vi "PH_Cam_BaseClass.save Image.vi"(0 "i ref in":refnum<vi>, 5 "error in (no error)":errorcluster) -> (14 "i ref out":refnum<vi>, 19 "error out":errorcluster)   [LabVIEW 2014, in "PH_Cam_BaseClass.lvlib"]
doc: "This CI saves the cam image if it finds a valid file refnum in own attributes."
uses:
  PH_Cam_BaseClass.lvlib
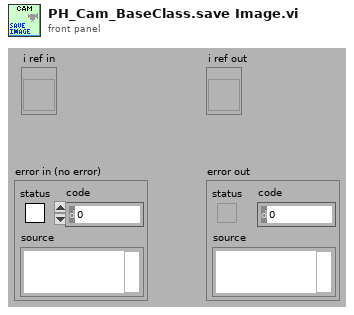
[diagram p1: front panel]
types:
  T1 = typedef "PH_Cam_BaseClass.lvlib/PH_Cam_BaseClass.i attribute.ctl" = cluster{"Gui Refs":T2, "Cam":cluster{"Source Notifier":refnum<notifier>, "Error":errorcluster, "Camera ID":string}, "Images":cluster{"Cam":T3, "Operation":T3, "PSDB":T3}, "Window Image":cluster{"Indicate Image":bool, "Window No.":i32, "Scale Facor":dbl, "Center Cross":bool, "Subtract Backgr":bool, "CoG":bool, "Color Palette":cluster{"Red":u8, "Green":u8, "Blue":u8}[], "Image On":bool}, "Default Prdc Int":i32, "Performance":cluster{"on":bool, "Timestamp Last Frame":i32}, "Histogram":cluster{"on":bool, "Mapping":bool}, "Save Image":cluster{"Save":bool, "File refnum":refnum<file>}, "Setting Service ID":i32, "Screen":cluster{"x-resolution":i16, "y-resolution":i16}, "On":bool, "Constructor finished":bool, "configured":bool}
  T2 = typedef "PH_Cam_BaseClass.lvlib/PH_Cam_BaseClass.GUI Refs.ctl" = cluster{"Frame Rate":refnum<vi>, "Get Frame Rate":refnum<vi>, "Show Image":refnum<vi>, "Get Histogram":refnum<vi>, "Mapping":refnum<vi>, "Histogram":refnum<vi>, "Center Cross":refnum<vi>, "Center of Gravity":refnum<vi>, "Scale Factor [%]":refnum<vi>, "Save Image":refnum<vi>, "Palette":refnum<vi>, "Subtract Background":refnum<vi>, "Cam Error":refnum<vi>, "On":refnum<vi>, "Cam List":refnum<vi>}
  T3 = typedef "IMAQ Image.ctl" = refnum<image>
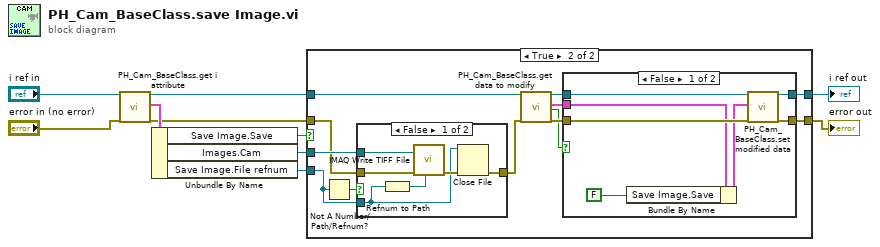
[diagram p0: block diagram]
diagram:
  n1 = call "PH_Cam_BaseClass.get i attribute.vi"("i ref in"="i ref in", "error in (no error)"="error in (no error)") -> ("i ref out"=w2:refnum<vi>, "i attribute"=w9:T1, "error out"=w6:errorcluster)  [unwired: 15 in]
  n2 = Unbundle By Name(w9) -> ("Save Image.Save"=w3:bool, "Images.Cam"=w8:T3, "Save Image.File refnum"=w4:refnum<file>)
  n3 = case shown="True" w3 {
    tunnel: [w11 w16] -> w10
    tunnel: w8 -> [_ w22]
    tunnel: w6 -> [w11 w13]
    tunnel: w4 -> [_ w23]
    tunnel: w2 -> [w12 w21]
    tunnel: [w12 w18] -> w1
    frame False {
    }
    frame True {
      n4 = Not A Number/Path/Refnum?(number/path/refnum=w23) -> (NaN/Path/Refnum?=w24:bool)
      n5 = case shown="False" w24 {
        tunnel: [w39 w40] -> w17
        tunnel: w13 -> [w37 w40]
        tunnel: w22 -> [w36 _]
        tunnel: w23 -> [w35 _]
        frame False {
          n6 = Refnum to Path(1:w35) -> (0:w34:path)
          n7 = call "IMAQ Write TIFF File"("error in (no error)"=w37, "File Path"=w34, "Image"=w36) -> ("error out"=w38:errorcluster)  [unwired: 5 in]
          n8 = Close File(refnum=w35, error in=w38) -> (error out=w39:errorcluster)  [unwired: 1 out]
        }
        frame True {
        }
      }
      n9 = call "PH_Cam_BaseClass.get data to modify.vi"("i ref in"=w21, "error in (no error)"=w17) -> ("i ref out"=w19:refnum<vi>, "i attribute"=w15:T1, "timed out"=w14:bool, "error out"=w20:errorcluster)  [unwired: 14 in]
      n10 = case shown="False" w14 {
        tunnel: w20 -> [w31 w32]
        tunnel: w19 -> [w30 w33]
        tunnel: [w29 w33] -> w18
        tunnel: [w28 w32] -> w16
        tunnel: w15 -> [w27 _]
        frame False {
          n11 = Bundle By Name(cluster=w27, "Save Image.Save"=FALSE) -> (w26:T1)
          n12 = call "PH_Cam_BaseClass.set modified data.vi"("i ref in"=w30, "i attribute"=w26, "error in (no error)"=w31) -> ("i ref out"=w29:refnum<vi>, "error out"=w28:errorcluster)  [unwired: 15 in]
        }
        frame True {
        }
      }
    }
  }
  "i ref out" <- w1
  "error out" <- w10
